vi "lsl append child value.vi"(8 "error in (no error)":errorcluster, 9 "value":string, 10 "name":string, 11 "xml_ptr":u64) -> (0 "error out":errorcluster, 2 "function return":u32, 3 "xml_ptr out":u64)   [LabVIEW 2016, in "Lab Streaming Layer.lvlib"]
doc: "extern LIBLSL_C_API lsl_xml_ptr lsl_append_child_value(lsl_xml_ptr e, const char *name, const char *value);"
uses:
  Lab Streaming Layer.lvlib
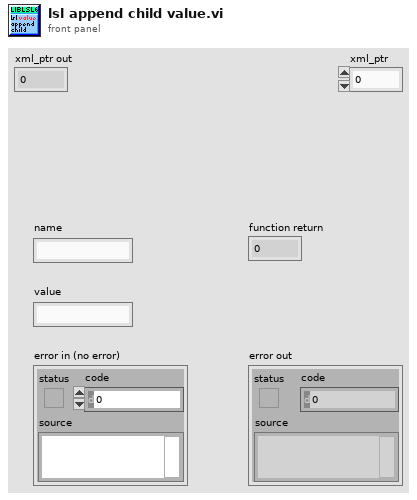
[diagram p1: front panel]
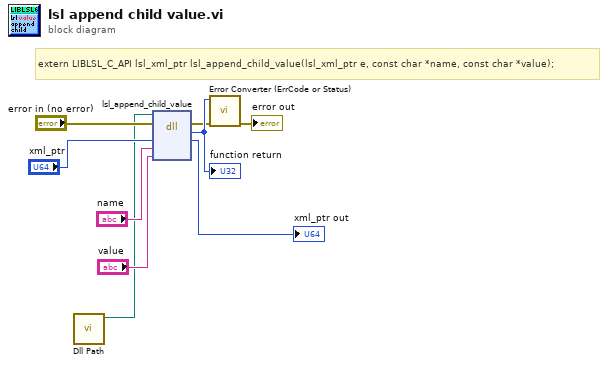
[diagram p0: block diagram]
diagram:
  # "extern LIBLSL_C_API lsl_xml_ptr lsl_append_child_value(lsl_xml_ptr e, const char *name, const char *value);"
  n1 = call "Dll Path.vi"() -> ("Dll path"=w1:path)  [unwired: 11 in]
  n2 = dll-call lib="E:/LabStreamingLayer/liblsl-LabVIEW-master/liblsl-LabVIEW-master/lsl.dll" fn="lsl_append_child_value"(path in=w1, error in="error in (no error)", "xml_ptr"="xml_ptr", "name"="name", "value"="value") -> (error out=w5:errorcluster, "return type"=w9:u32, "xml_ptr"=→"xml_ptr out":u64)  [unwired: 3 in, 1 out]
  "function return" <- w9
  n3 = call "Error Converter (ErrCode or Status).vi"("error in (no error)"=w5, "error code"=w9) -> ("error out"=→"error out":errorcluster)  [unwired: 9 in]
